vi "JuPyter Client Test.vi"() -> ()   [LabVIEW 2018]
doc: "A demonstration of a client application to communicate with a JuPyter kernel. \n\nThis client will atempt to discover a suitable ipython executable and invoke it as a kernel with a connection file. It can then communicate with the kernel, passing strings to it and collecting the results. \n\nTo help in seeing what is going on, the messages returned by the kernel are also displayed."
uses:
  Shell Messages/execute_request Message/User Expression.ctl
  IOPub Messages/status Message/Status Content.ctl
  Utility/Connection.ctl
  IOPub Messages/status Message/status Message.lvclass
  Shell Messages/kernel_info_reply Message/kernel_info_reply Message.lvclass
  IOPub Messages/error Message/error Message.lvclass
  Shell Messages/execute_reply Message/execute_reply Message.lvclass
  C:/Users/gavin/Documents/LabVIEW Data/LabVIEW-Bits/Connectivity/Jupyter Client/Base Classes/Reply Message/Reply Message.lvclass
  IOPub Messages/stream Message/stream Message.lvclass
  IOPub Messages/execute_result Message/execute_result Message.lvclass
  C:/Users/gavin/Documents/LabVIEW Data/LabVIEW-Bits/Connectivity/Jupyter Client/IOPub Messages/display_data Message/display_data Message.lvclass
  Shell Messages/shutdown_request Message/shutdown_request Message.lvclass
  Shell Messages/kernel_info_request Message/kernel_info_request Message.lvclass
  Shell Messages/execute_request Message/execute_request Message.lvclass
  48e361d1-6cf2-4824-8834-e089fd543d5e.vi
  48e361d1-6cf2-4824-8834-e089fd543d5e.vi/b5d30270-35b7-4a17-a433-2392ca8f7161.vi
  48e361d1-6cf2-4824-8834-e089fd543d5e.vi/d3509066-e9e6-4190-b64c-7d002659779e.vi
  48e361d1-6cf2-4824-8834-e089fd543d5e.vi/da8d85e9-ca35-4b20-8115-8457edcb746c.vi
  JuPyter_Client/public/Start Kernel and Connect.vi
  JuPyter_Client/public/Connect with Connection File.vi
  JuPyter_Client/public/Connect with Connection Cluster.vi
  <vilib>/JDP Science/JSONtext/Variant to JSON Text.vi
  <vilib>/JDP Science/JSONtext/Set Item.vi
  Base Classes/Message Class/Message Class.lvclass
  JuPyter_Client/JuPyter_Client.lvclass
  ClientMessaging.lvlib
panel:
  in  "Outputs":T1(tab)
  in  "Connection JSON":string
  in  "Connect to kernel":bool
  in  "Connection Method":T2(ring)
  in  "Path to Kernel Command (IPython)":string="\n" caption="Path to Kernel Command (IPython) - blank to search"
  in  "Connection Info":T3
  in  "Connection File (default=guess)":path
  in  "Streams":enum32{"stdout", "stdeerr"}(tab)
  in  "Cl;ear stdout":bool
  out "Stdout":string
  in  "Cl;ear stderr":bool
  out "stderr":string
  in  "Clear Results":bool
  out "Results":string[](array[string])
  in  "Clear Message":bool
  out "Message Data":string
  in  "Variables to Watch":T4[](array[typedef])
  out "Client Error State":errorcluster
  in  "Enter":bool
  in  "Code":string
  in  "Exit":bool
  out "Heartbeat":bool
  out "Language and Version":string
  out "status":T5
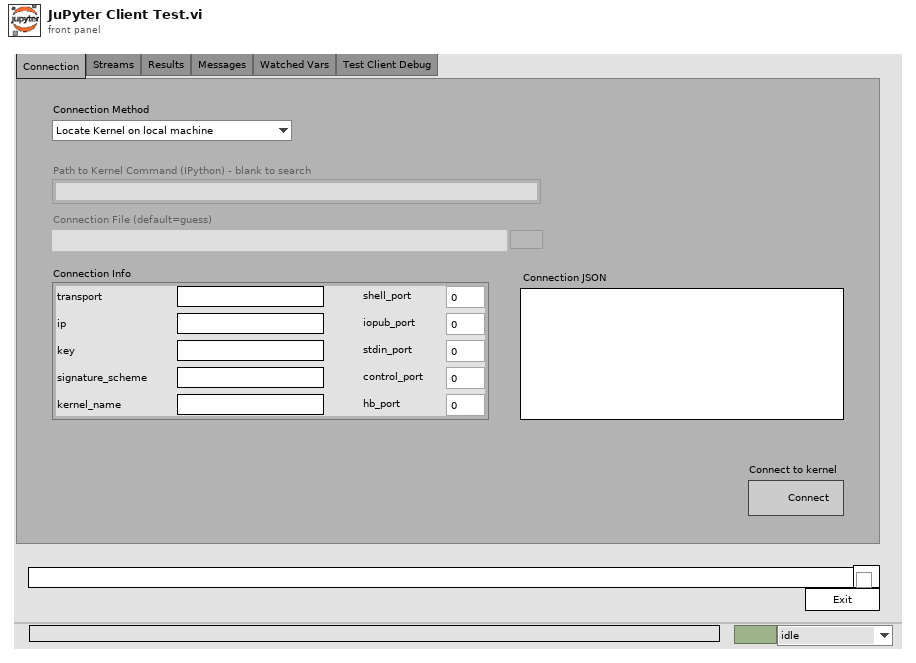
[diagram p1: front panel]
types:
  T1 = enum32{"Connection", "Streams", "Results", "Messages", "Watched Vars", "Test Client Debug"}
  T2 = enum16{"Locate Kernel on local machine", "Provide path to connection file", "Set connection details manually"}
  T3 = typedef "ClientMessaging.lvlib/Connection.ctl" = cluster{"transport":string, "ip":string, "key":string, "signature_scheme":string, "kernel_name":string, "shell_port":u16, "iopub_port":u16, "stdin_port":u16, "control_port":u16, "hb_port":u16}
  T4 = typedef "ClientMessaging.lvlib/execute_reply Message.lvclass/User Expression.ctl" = cluster{"Variable":string, "Value":string, "Valid":bool}
  T5 = typedef "ClientMessaging.lvlib/status Message.lvclass/Status Content.ctl" = enum16{"idle", "busy", "starting"}
  T6 = typedef "ClientMessaging.lvlib/Message Class.lvclass/header_dict.ctl" = cluster{"msg_id":string, "username":string, "session":string, "date":timestamp, "msg_type":string, "version":string}
  T7 = cluster{"ename":string, "evalue":string, "traceback":string[]}
  T8 = typedef "User Expression.ctl" = cluster{"Variable":string, "Value":string, "Valid":bool}
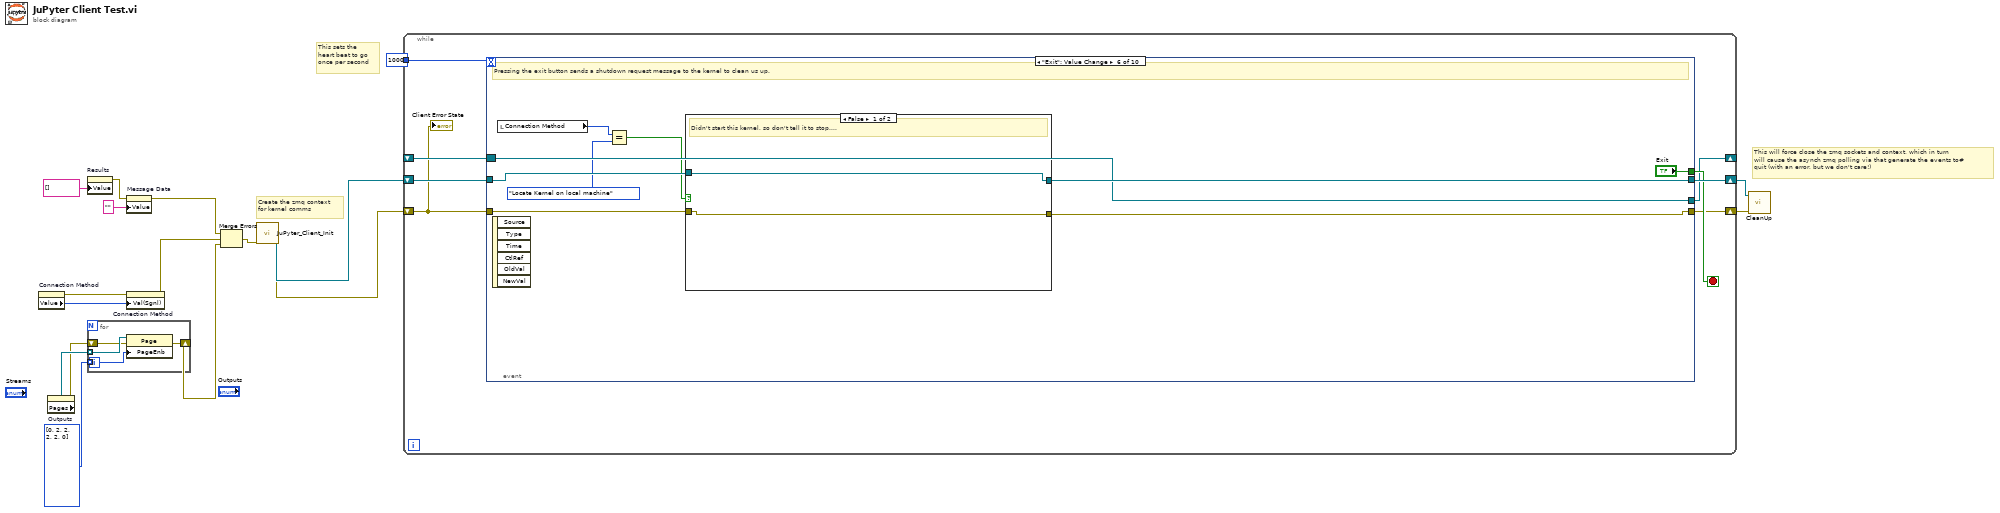
[diagram p0: block diagram]
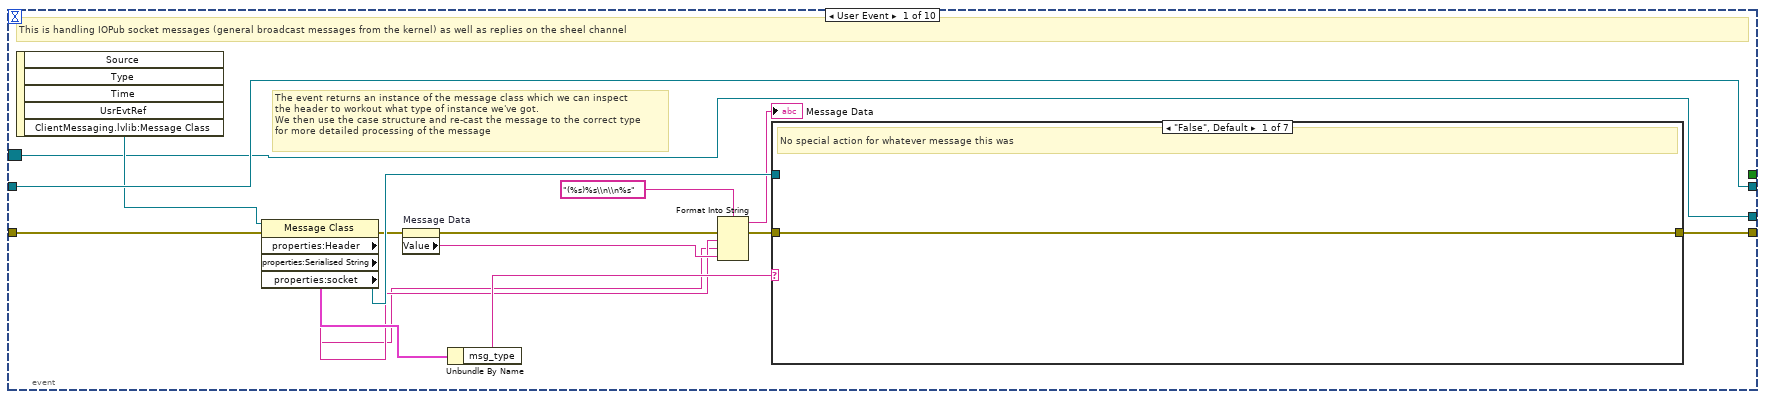
[diagram p2: hidden frame]
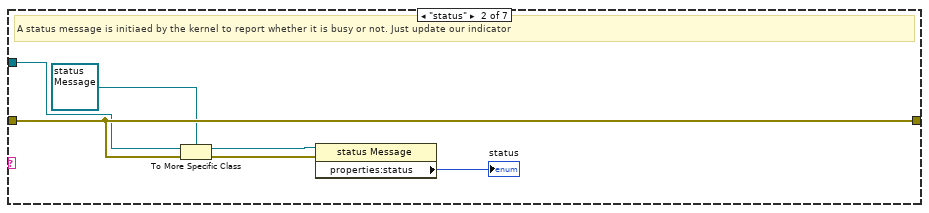
[diagram p3: hidden frame]
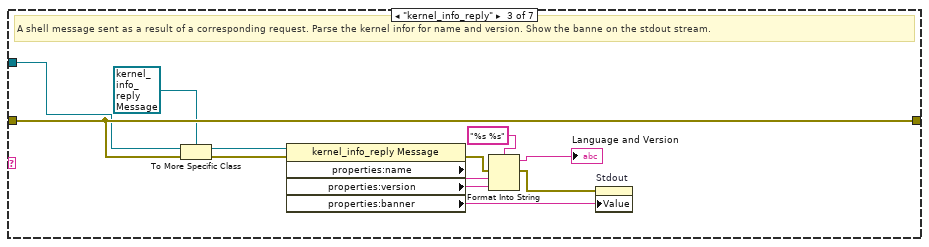
[diagram p4: hidden frame]
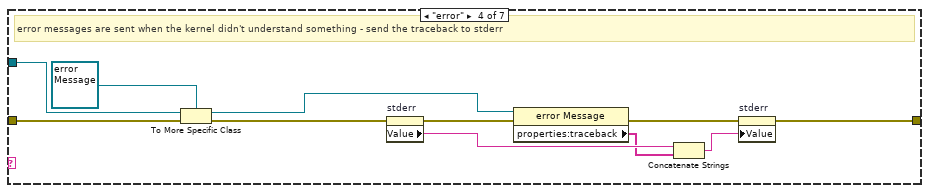
[diagram p5: hidden frame]
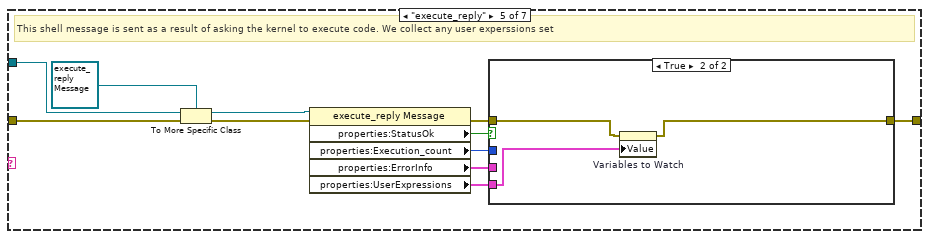
[diagram p6: hidden frame]
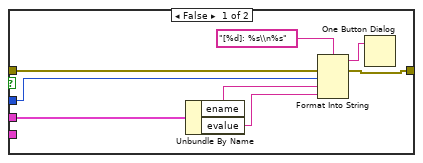
[diagram p7: hidden frame]
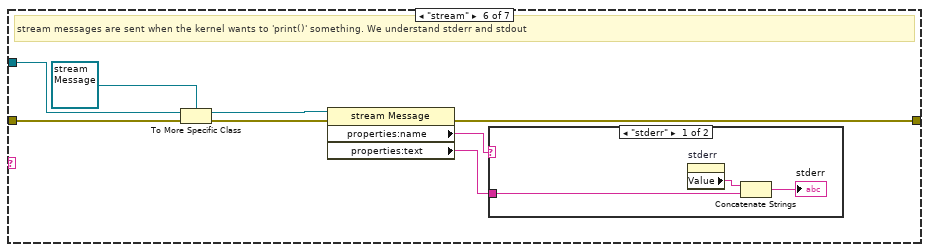
[diagram p8: hidden frame]
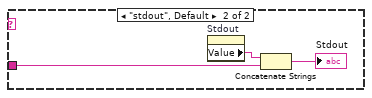
[diagram p9: hidden frame]
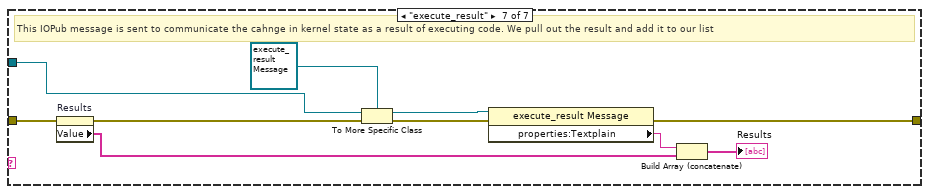
[diagram p10: hidden frame]
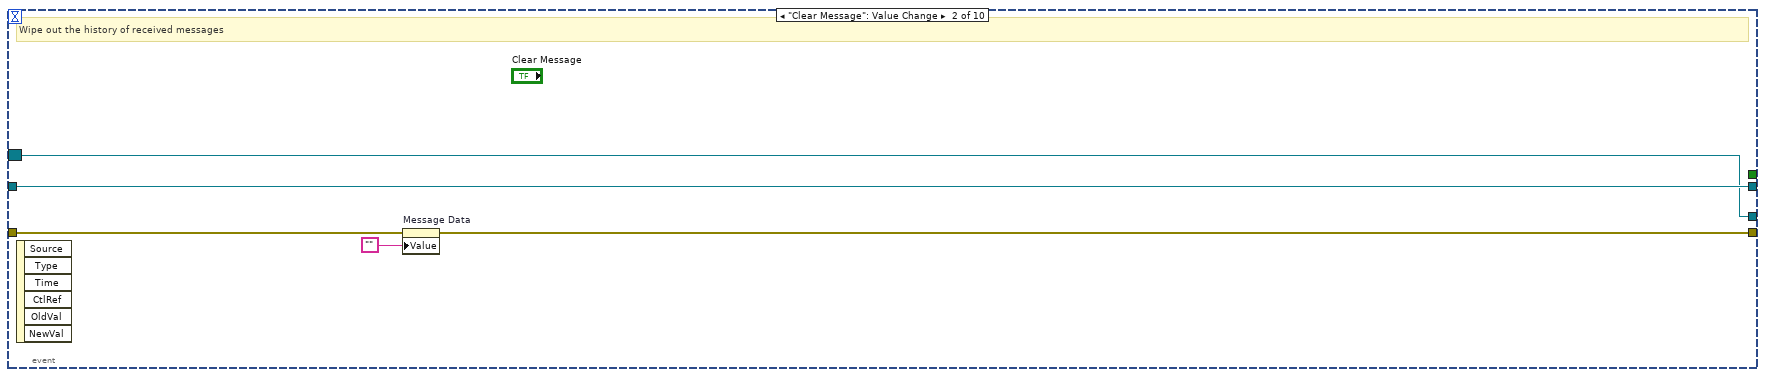
[diagram p11: hidden frame]
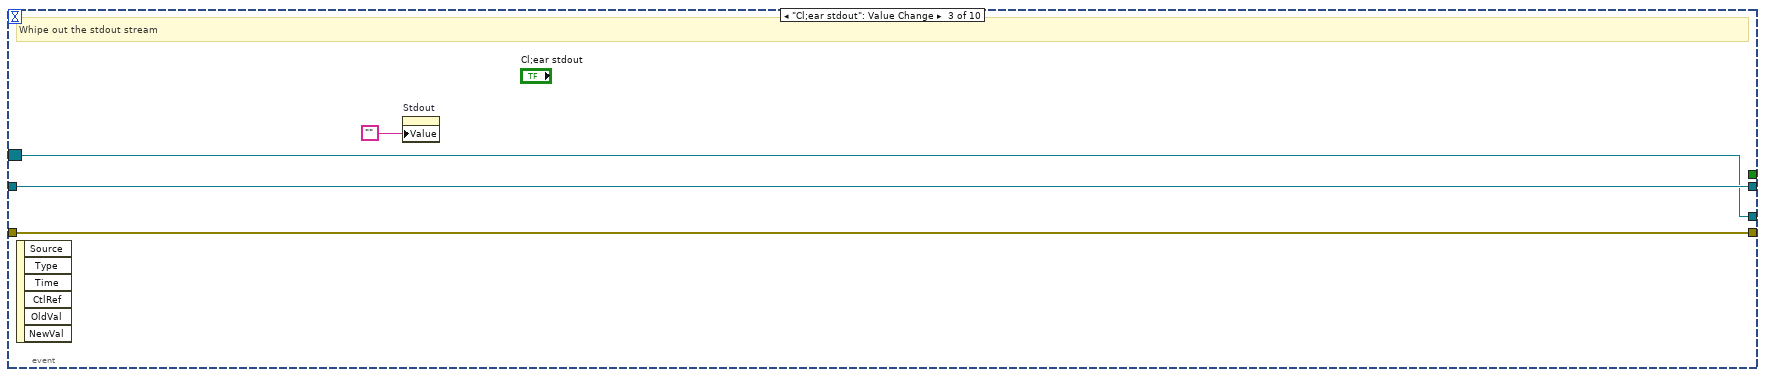
[diagram p12: hidden frame]
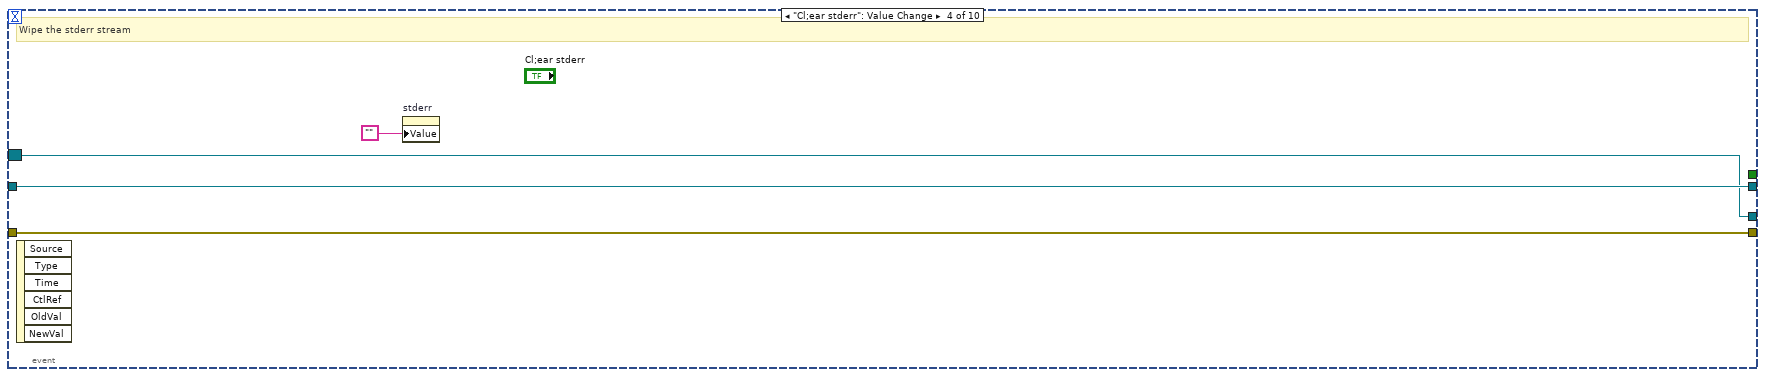
[diagram p13: hidden frame]
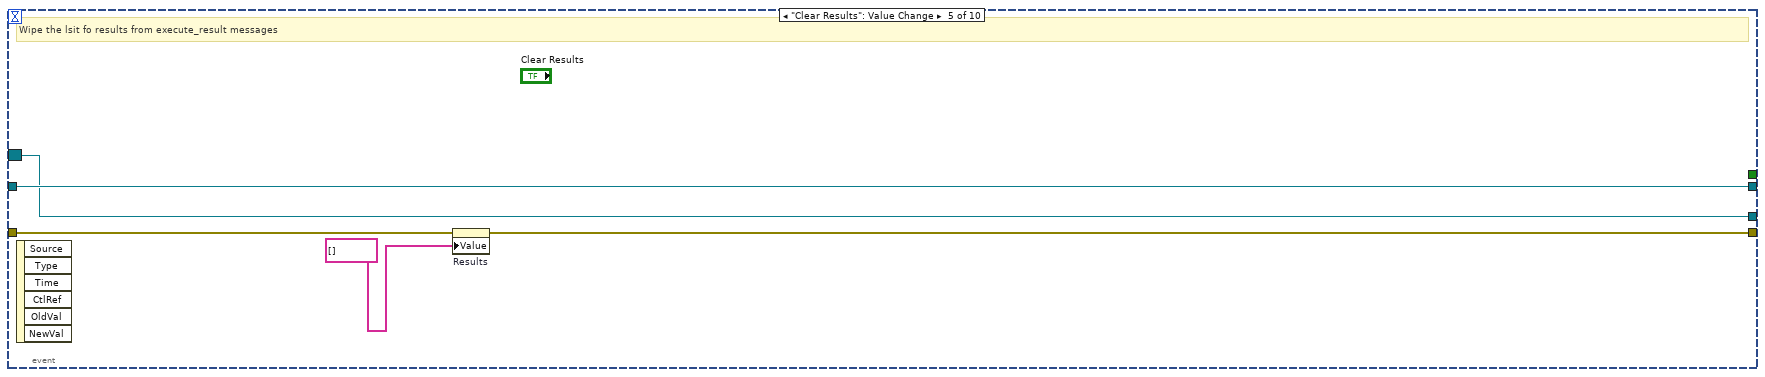
[diagram p14: hidden frame]
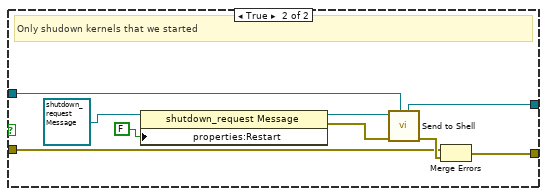
[diagram p15: hidden frame]
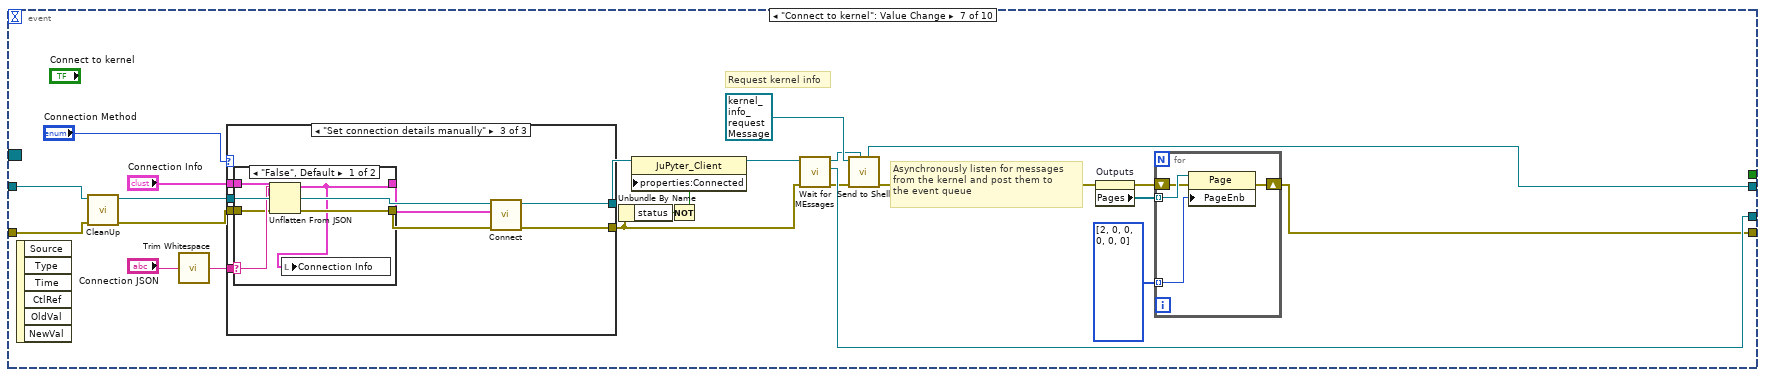
[diagram p16: hidden frame]
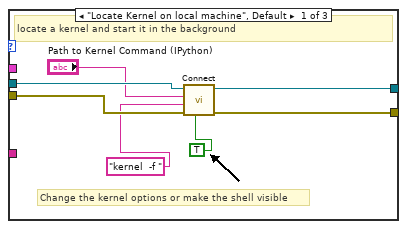
[diagram p17: hidden frame]
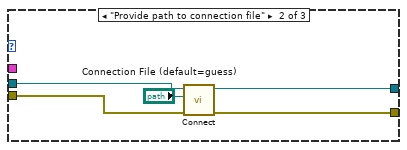
[diagram p18: hidden frame]
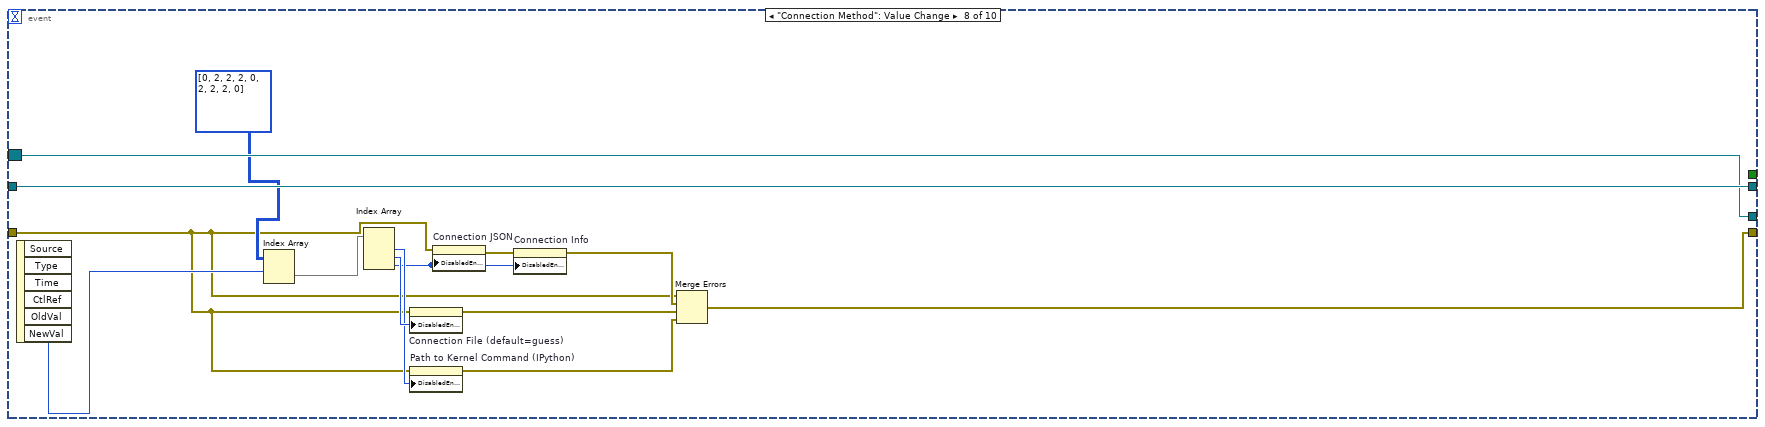
[diagram p20: hidden frame]
diagram:
  # "This sets the\nheart beat to go\nonce per second"
  # "This will force close the zmq sockets and context, which in turn\nwill cause the asynch zmq polling via that generate the events to#\nquit (with an error, but we don't care!)"
  # "Create the zmq context\nfor kernel comms"
  n1 = property on="Connection Method" class="Enum (strict)"() -> (error out=w8:errorcluster, "Value"=w7:T2)  [unwired: 2 in, 1 out]
  n2 = property on="Outputs" class="TabCtl (strict)"() -> (error out=w3:errorcluster, "Pages"=w4:refnum<vi>[])  [unwired: 2 in, 1 out]
  n3 = property on="Results" class="Arr (strict)"("Value"=string[] [] ("Results")) -> (error out=w13:errorcluster)  [unwired: 2 in, 1 out]
  n4 = for {
    tunnel: w4 -> [w21] mode=indexing
    shift-right: [w19] -> w1
    shift-left: w3 -> [w20]
    tunnel: i32[] [0, 2, 2, 2, 2, 0] -> [w18] mode=indexing
    n5 = property class="Page"(reference=w21, error in=w20, "PageEnb"=w18) -> (error out=w19:errorcluster)  [unwired: 1 out]
  }
  n6 = property on="Message Data" class="Str"(error in=w13, "Value"="" ("Message Data")) -> (error out=w14:errorcluster)  [unwired: 1 in, 1 out]
  n7 = property on="Connection Method" class="Enum (strict)"(error in=w8, "Val(Sgnl)"=w7) -> (error out=w5:errorcluster)  [unwired: 1 in, 1 out]
  n8 = Merge Errors(w14, w5, w1) -> (w6:errorcluster)
  n9 = call "JuPyter_Client_Init.vi"("error in (no error)"=w6) -> ("error out"=w9:errorcluster, "object out"=w10:refnum<class "JuPyter_Client.lvclass">)  [unwired: 9 in]
  n10 = while {
    shift-right: [w29] -> w17
    shift-left: w10 -> [w26]
    shift-right: [w27] -> w16
    shift-left: w9 -> [w23]
    tunnel: 1000 -> [w24]
    shift-right: [w22] -> _
    shift-left: _ -> [w25]
    stop <- w28 stop-if-true
    n11 = event shown="[5] \"Exit\": Value Change" {
      selector: w25 -> [w30 w122 w127 w131 w135 w143 _ w226 w228 w250]
      dyn-events: _ -> [_ _ _ _ _ _ _ _ _ _]
      timeout: w24 -> [_ _ _ _ _ _ _ _ _ _]
      tunnel: w23 -> [w37 w124 w129 w133 w137 w144 w182 w216 w233 w247]
      tunnel: [w43 w126 w130 w134 w139 w146 w173 w227 w239 w251] -> w29
      tunnel: [_ _ _ _ _ "Exit" _ _ _ w253] -> w28
      tunnel: [w44 w123 w129 w133 w136 w145 w167 w221 w236 w252] -> w27
      tunnel: w26 -> [w43 w126 w130 w134 w139 w147 w181 w227 w238 w254]
      tunnel: [w30 w122 w127 w131 w135 w143 w176 w226 w228 w250] -> w22
      event User Event {
        # "The event returns an instance of the message class which we can inspect\nthe header to workout what type of instance we've got.\nWe then use the case structure and re-cast the message to the correct type\nfor more detailed processing of the message"
        # "This is handling IOPub socket messages (general broadcast messages from the kernel) as well as replies on the sheel channel"
        n12 = event-data() -> ("ClientMessaging.lvlib:Message Class"=w38:refnum<class "Message Class.lvclass">)  [unwired: 1 in, 4 out]
        n13 = property class="Message Class"(reference=w38, error in=w37) -> (reference out=w42:refnum<class "Message Class.lvclass">, error out=w35:errorcluster, "properties:Header"=w41:T6, "properties:Serialised String"=w31:string, "properties:socket"=w32:string)
        n14 = property on="Message Data" class="Str"(error in=w35) -> (error out=w34:errorcluster, "Value"=w33:string)  [unwired: 1 in, 1 out]
        n15 = Unbundle By Name(w41) -> ("msg_type"=w45:string)
        n16 = Format Into String(format string="(%s)%s\\n\\n%s", error in=w34, w32, w31, w33) -> (resulting string=→"Message Data":string, error out=w36:errorcluster)  [unwired: 1 in]
        n17 = case shown="\"False\", Default" w45 {
          tunnel: w42 -> [_ w50 w63 w74 w85 w105 w120]
          tunnel: w36 -> [w46 w52 w64 w75 w86 w103 w113]
          tunnel: [w46 w52 w64 w65 w77 w100 w121] -> w44
          frame "False", Default {
            # "No special action for whatever message this was"
          }
          frame "status" {
            # "A status message is initiaed by the kernel to report whether it is busy or not. Just update our indicator"
            n18 = To More Specific Class(target class=refnum<class "status Message.lvclass"> refnum ("ClientMessaging.lvlib:status Message"), reference=w50, error in=w52) -> (specific class reference=w49:refnum<class "status Message.lvclass">, error out=w48:errorcluster)
            n19 = property class="status Message"(reference=w49, error in=w48) -> ("properties:status"=→"status":T5)  [unwired: 2 out]
          }
          frame "kernel_info_reply" {
            # "A shell message sent as a result of a corresponding request. Parse the kernel infor for name and version. Show the banne on the stdout stream."
            n20 = To More Specific Class(target class=refnum<class "kernel_info_reply Message.lvclass"> refnum ("ClientMessaging.lvlib:kernel_info_reply"), reference=w63, error in=w64) -> (specific class reference=w62:refnum<class "kernel_info_reply Message.lvclass">, error out=w61:errorcluster)
            n21 = property class="kernel_info_reply Message"(reference=w62, error in=w61) -> (error out=w58:errorcluster, "properties:name"=w57:string, "properties:version"=w56:string, "properties:banner"=w53:string)  [unwired: 1 out]
            n22 = Format Into String(format string="%s %s", error in=w58, w57, w56) -> (resulting string=→"Language and Version":string, error out=w54:errorcluster)  [unwired: 1 in]
            n23 = property on="Stdout" class="Str"(error in=w54, "Value"=w53) -> ()  [unwired: 1 in, 2 out]
          }
          frame "error" {
            # "error messages are sent when the kernel didn't understand something - send the traceback to stderr"
            n24 = To More Specific Class(target class=refnum<class "error Message.lvclass"> refnum ("ClientMessaging.lvlib:error Message"), reference=w74, error in=w75) -> (specific class reference=w73:refnum<class "error Message.lvclass">, error out=w68:errorcluster)
            n25 = property on="stderr" class="Str"(error in=w68) -> (error out=w67:errorcluster, "Value"=w71:string)  [unwired: 1 in, 1 out]
            n26 = property class="error Message"(reference=w73, error in=w67) -> (error out=w66:errorcluster, "properties:traceback"=w70:string[])  [unwired: 1 out]
            n27 = Concatenate Strings(w71, w70) -> (w69:string)
            n28 = property on="stderr" class="Str"(error in=w66, "Value"=w69) -> (error out=w65:errorcluster)  [unwired: 1 in, 1 out]
          }
          frame "execute_reply" {
            # "This shell message is sent as a result of asking the kernel to execute code. We collect any user experssions set"
            n29 = To More Specific Class(target class=refnum<class "execute_reply Message.lvclass"> refnum ("ClientMessaging.lvlib:execute_reply Message"), reference=w85, error in=w86) -> (specific class reference=w84:refnum<class "execute_reply Message.lvclass">, error out=w79:errorcluster)
            n30 = property class="execute_reply Message"(reference=w84, error in=w79) -> (error out=w78:errorcluster, "properties:StatusOk"=w82:bool, "properties:Execution_count"=w81:u32, "properties:ErrorInfo"=w80:T7, "properties:UserExpressions"=w76:T8[])  [unwired: 1 out]
            n31 = case shown="True" w82 {
              tunnel: w81 -> [w92 _]
              tunnel: w80 -> [w94 _]
              tunnel: w78 -> [w88 w96]
              tunnel: [w87 w95] -> w77
              tunnel: w76 -> [_ w97]
              frame False {
                n32 = Unbundle By Name(w94) -> ("ename"=w91:string, "evalue"=w90:string)
                n33 = Format Into String(format string="[%d]: %s\\n%s", error in=w88, w92, w91, w90) -> (resulting string=w89:string, error out=w87:errorcluster)  [unwired: 1 in]
                n34 = One Button Dialog(message=w89) -> ()  [unwired: 1 in, 1 out]
              }
              frame True {
                n35 = property on="Variables to Watch" class="Arr (strict)"(error in=w96, "Value"=w97) -> (error out=w95:errorcluster)  [unwired: 1 in, 1 out]
              }
            }
          }
          frame "stream" {
            # "stream messages are sent when the kernel wants to 'print()' something. We understand stderr and stdout"
            n36 = To More Specific Class(target class=refnum<class "stream Message.lvclass"> refnum ("ClientMessaging.lvlib:stream Message"), reference=w105, error in=w103) -> (specific class reference=w102:refnum<class "stream Message.lvclass">, error out=w101:errorcluster)
            n37 = property class="stream Message"(reference=w102, error in=w101) -> (error out=w100:errorcluster, "properties:name"=w99:string, "properties:text"=w98:string)  [unwired: 1 out]
            n38 = case shown="\"stderr\"" w99 {
              tunnel: w98 -> [w107 w110]
              frame "stderr" {
                n39 = property on="stderr" class="Str"() -> ("Value"=w108:string)  [unwired: 2 in, 2 out]
                n40 = Concatenate Strings(w108, w107) -> (→"stderr":string)
              }
              frame "stdout", Default {
                n41 = property on="Stdout" class="Str"() -> ("Value"=w111:string)  [unwired: 2 in, 2 out]
                n42 = Concatenate Strings(w111, w110) -> (→"Stdout":string)
              }
            }
          }
          frame "execute_result" {
            # "This IOPub message is sent to communicate the cahnge in kernel state as a result of executing code. We pull out the result and add it to our list"
            n43 = property on="Results" class="Arr (strict)"(error in=w113) -> (error out=w112:errorcluster, "Value"=w114:string[])  [unwired: 1 in, 1 out]
            n44 = To More Specific Class(target class=refnum<class "execute_result Message.lvclass"> refnum ("ClientMessaging.lvlib:execute_result Message"), reference=w120, error in=w112) -> (specific class reference=w118:refnum<class "execute_result Message.lvclass">, error out=w117:errorcluster)
            n45 = property class="execute_result Message"(reference=w118, error in=w117) -> (error out=w121:errorcluster, "properties:Textplain"=w116:string)  [unwired: 1 out]
            n46 = Build Array (concatenate)(w116, w114) -> (→"Results":string[])
          }
        }
      }
      event "Clear Message": Value Change {
        # "Wipe out the history of received messages"
        n47 = event-data() -> ()  [unwired: 1 in, 6 out]
        n48 = property on="Message Data" class="Str"(error in=w124, "Value"="") -> (error out=w123:errorcluster)  [unwired: 1 in, 1 out]
      }
      event "Cl;ear stdout": Value Change {
        # "Whipe out the stdout stream"
        n49 = event-data() -> ()  [unwired: 1 in, 6 out]
        n50 = property on="Stdout" class="Str"("Value"="") -> ()  [unwired: 2 in, 2 out]
      }
      event "Cl;ear stderr": Value Change {
        # "Wipe the stderr stream"
        n51 = event-data() -> ()  [unwired: 1 in, 6 out]
        n52 = property on="stderr" class="Str"("Value"="") -> ()  [unwired: 2 in, 2 out]
      }
      event "Clear Results": Value Change {
        # "Wipe the lsit fo results from execute_result messages"
        n53 = event-data() -> ()  [unwired: 1 in, 6 out]
        n54 = property on="Results" class="Arr (strict)"(error in=w137, "Value"=string[] [] ("Results")) -> (error out=w136:errorcluster)  [unwired: 1 in, 1 out]
      }
      event "Exit": Value Change {
        # "Pressing the exit button sends a shutdown request message to the kernel to clean us up."
        n55 = event-data() -> ()  [unwired: 1 in, 6 out]
        n56 = local read "Connection Method"() -> (w142:T2)
        n57 = Equal?(x=w142, y=T2."Locate Kernel on local machine") -> (x = y?=w140:bool)
        n58 = case shown="False" w140 {
          tunnel: w147 -> [w150 w158]
          tunnel: [w150 w157] -> w146
          tunnel: [w149 w152] -> w145
          tunnel: w144 -> [w149 w151]
          frame False {
            # "Didn't start this kernel, so don't tell it to stop...."
          }
          frame True {
            # "Only shudown kernels that we started"
            n59 = property class="shutdown_request Message"(reference=refnum<class "shutdown_request Message.lvclass"> refnum ("ClientMessaging.lvlib:shutdown_request Message"), "properties:Restart"=FALSE ("Restart")) -> (reference out=w155:refnum<class "shutdown_request Message.lvclass">, error out=w154:errorcluster)  [unwired: 1 in]
            n60 = call-dynamic "Send to Shell.vi"("Session In"=w158, "error in (no error)"=w154, "object in"=w155) -> ("error out"=w156:errorcluster, "Session Out"=w157:refnum<class "JuPyter_Client.lvclass">)  [unwired: 5 in, 2 out]
            n61 = Merge Errors(w151, w156) -> (w152:errorcluster)
          }
        }
      }
      event "Connect to kernel": Value Change {
        # "Asynchronously listen for messages\nfrom the kernel and post them to\nthe event queue"
        # "Request kernel info"
        n62 = event-data() -> ()  [unwired: 1 in, 6 out]
        n63 = call-dynamic "CleanUp.vi"("error in (no error)"=w182, "object in"=w181) -> ("error out"=w178:errorcluster, "object out"=w179:refnum<class "JuPyter_Client.lvclass">)  [unwired: 8 in]
        n64 = call <vilib>:"Trim Whitespace.vi"("string"="Connection JSON") -> ("trimmed string"=w160:string)  [unwired: 1 in]
        n65 = case shown="\"Set connection details manually\"" "Connection Method" {
          tunnel: w179 -> [w193 w198 w206]
          tunnel: w178 -> [w192 w197 w199]
          tunnel: [w190 w196 w205] -> w177
          tunnel: [w189 w195 w204] -> w165
          tunnel: "Connection Info" -> [_ _ w201]
          tunnel: w160 -> [_ _ w203]
          frame "Locate Kernel on local machine", Default {
            # "Change the kernel options or make the shell visible"
            # "locate a kernel and start it in the background"
            n66 = call-poly "Connect.vi"("run minimized? (F)"=TRUE, "error in (no error)"=w192, "args"="kernel  -f ", "Path to Kernel Command (IPython)"="Path to Kernel Command (IPython)", "object in"=w193) -> ("error out"=w189:errorcluster, "object out"=w190:refnum<class "JuPyter_Client.lvclass">)  [unwired: 5 in]
          }
          frame "Provide path to connection file" {
            n67 = call-poly "Connect.vi"("error in (no error)"=w197, "Connection File (default=guess)"="Connection File (default=guess)", "object in"=w198) -> ("error out"=w195:errorcluster, "object out"=w196:refnum<class "JuPyter_Client.lvclass">)  [unwired: 7 in]
          }
          frame "Set connection details manually" {
            n68 = case shown="\"False\", Default" w203 {
              selector: w203 -> [w211 _]
              tunnel: [w207 w213] -> w202
              tunnel: w201 -> [w210 w213]
              tunnel: [w208 w212] -> w200
              tunnel: w199 -> [w209 w212]
              frame "False", Default {
                n69 = Unflatten From JSON(JSON string=w211, type and defaults=w210, error in (no error)=w209) -> (value=w207:T3, error out=w208:errorcluster)  [unwired: 4 in]
                n70 = local write "Connection Info"(w207) -> ()
              }
              frame "\u0000" {
              }
            }
            n71 = call-poly "Connect.vi"("error in (no error)"=w200, "Connection Info"=w202, "object in"=w206) -> ("error out"=w204:errorcluster, "object out"=w205:refnum<class "JuPyter_Client.lvclass">)  [unwired: 7 in]
          }
        }
        n72 = Unbundle By Name(w165) -> ("status"=w164:bool)
        n73 = Not(x=w164) -> (.not. x?=w163:bool)
        n74 = property class="JuPyter_Client"(reference=w177, "properties:Connected"=w163) -> (reference out=w166:refnum<class "JuPyter_Client.lvclass">)  [unwired: 1 in, 1 out]
        n75 = call-dynamic "Wait for MEssages.vi"("error in (no error)"=w165, "object in"=w166) -> ("error out"=w172:errorcluster, "Event Registration Refnum"=w176:refnum<event-registration>, "object out"=w174:refnum<class "JuPyter_Client.lvclass">)  [unwired: 7 in]
        n76 = call-dynamic "Send to Shell.vi"("Session In"=w174, "error in (no error)"=w172, "object in"=refnum<class "kernel_info_request Message.lvclass"> refnum ("ClientMessaging.lvlib:kernel_info_request Message")) -> ("error out"=w168:errorcluster, "Session Out"=w173:refnum<class "JuPyter_Client.lvclass">)  [unwired: 5 in, 2 out]
        n77 = property on="Outputs" class="TabCtl (strict)"(error in=w168) -> (error out=w170:errorcluster, "Pages"=w169:refnum<vi>[])  [unwired: 1 in, 1 out]
        n78 = for {
          tunnel: w169 -> [w186] mode=indexing
          shift-right: [w184] -> w167
          shift-left: w170 -> [w185]
          tunnel: i32[] [2, 0, 0, 0, 0, 0] -> [w183] mode=indexing
          n79 = property class="Page"(reference=w186, error in=w185, "PageEnb"=w183) -> (error out=w184:errorcluster)  [unwired: 1 out]
        }
      }
      event "Connection Method": Value Change {
        n80 = event-data() -> ("NewVal"=w225:T2)  [unwired: 1 in, 5 out]
        n81 = Index Array(array=i32[][] [[0, 2, 2], [2, 0, 2], [2, 2, 0]], index (row)=w225) -> (element=w223:i32[])  [unwired: 1 in]
        n82 = Index Array(array=w223) -> (element #1=w217:i32, element #2=w222:i32, element #3=w214:i32)  [unwired: 3 in]
        n83 = property on="Connection File (default=guess)" class="Path"(error in=w216, "DisabledEnum"=w222) -> (error out=w219:errorcluster)  [unwired: 1 in, 1 out]
        n84 = property on="Path to Kernel Command (IPython)" class="Str"(error in=w216, "DisabledEnum"=w217) -> (error out=w218:errorcluster)  [unwired: 1 in, 1 out]
        n85 = property on="Connection JSON" class="Str"(error in=w216, "DisabledEnum"=w214) -> (error out=w215:errorcluster)  [unwired: 1 in, 1 out]
        n86 = property on="Connection Info" class="Clust (strict)"(error in=w215, "DisabledEnum"=w214) -> (error out=w220:errorcluster)  [unwired: 1 in, 1 out]
        n87 = Merge Errors(w216, w220, w219, w218) -> (w221:errorcluster)
      }
      event "Enter": Value Change {
        # "Pressing enter  sends the string the user typeed as an execute_request message to the kernel"
        n88 = event-data() -> ()  [unwired: 1 in, 6 out]
        n89 = for {
          tunnel: "Variables to Watch" -> [w245] mode=indexing
          tunnel: [w244] -> w229 mode=indexing
          n90 = Unbundle By Name(w245) -> ("Variable"=w244:string)
        }
        n91 = call "Build User Expressions.vim"("error in (no error)"=w233, "List of variables to return"=w229, "object in"=refnum<class "execute_request Message.lvclass"> refnum ("ClientMessaging.lvlib:execute_request Message")) -> ("error out"=w234:errorcluster, "object out"=w235:refnum<class "execute_request Message.lvclass">)  [unwired: 7 in]
        n92 = property class="execute_request Message"(reference=w235, error in=w234, "properties:Code"="Code") -> (reference out=w241:refnum<class "execute_request Message.lvclass">, error out=w240:errorcluster)
        n93 = call-dynamic "Send to Shell.vi"("Session In"=w238, "error in (no error)"=w240, "object in"=w241) -> ("error out"=w231:errorcluster, "Session Out"=w239:refnum<class "JuPyter_Client.lvclass">)  [unwired: 5 in, 2 out]
        n94 = property on="Code" class="Str"(error in=w231, "Value"="" ("Code"), "Key Focus"=TRUE) -> (error out=w236:errorcluster)  [unwired: 1 in, 1 out]
      }
      event Timeout {
        # "Check the heartbeat by sending a byte on the heartbeat channel and wait for a response."
        n95 = event-data() -> ()  [unwired: 1 in, 3 out]
        n96 = property class="JuPyter_Client"(reference=w254, error in=w247) -> (reference out=w249:refnum<class "JuPyter_Client.lvclass">, error out=w246:errorcluster, "properties:Connected"=w248:bool)
        n97 = case shown="True" w248 {
          tunnel: w249 -> [w257 w263]
          tunnel: w246 -> [w256 w262]
          tunnel: [FALSE ("Timed out/error") w261] -> w253
          tunnel: [w256 w259] -> w252
          tunnel: [w257 w258] -> w251
          frame False {
          }
          frame True {
            n98 = call-dynamic "Check Heartbeat.vi"("error in (no error)"=w262, "object in"=w263) -> ("error out"=w260:errorcluster, "Timed out/error"=w261:bool, "object out"=w258:refnum<class "JuPyter_Client.lvclass">)  [unwired: 7 in]
            n99 = case shown="False" w261 {
              tunnel: w260 -> [w265 w268]
              tunnel: [w264 w268] -> w259
              frame False {
                # "Toggle the indicator"
                n100 = property on="Heartbeat" class="Bool (strict)"(error in=w265) -> (error out=w264:errorcluster, "Value"=w267:bool)  [unwired: 1 in, 1 out]
                n101 = Not(x=w267) -> (.not. x?=→"Heartbeat":bool)
              }
              frame True {
                # "Dead kernel !"
              }
            }
          }
        }
      }
    }
    "Client Error State" <- w23
  }
  n102 = call-dynamic "CleanUp.vi"("error in (no error)"=w16, "object in"=w17) -> ()  [unwired: 8 in, 2 out]
